vi "class_data.vi"() -> ()   [LabVIEW 2010, in "GenericInstrument.lvclass"]
uses:
  GenericInstrument.lvclass
panel:
  in  "latest instance":refnum<class "GenericInstrument.lvclass">
  in  "locked by":string
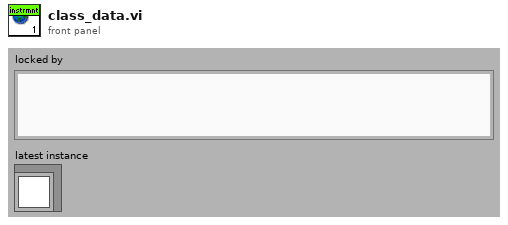
[diagram p1: front panel]
diagram:
